vi "ReceiveConnectionStatus.vi"(8 "error in (no error)":errorcluster, 11 "body":variant) -> (0 "error out":errorcluster, 1 "error code":i32, 3 "status":T1, 4 "error info":string)   [LabVIEW 2017, in "ServerComm.lvlib"]
doc: "Returns whether the connection between the device and NI InsightCM Server is online or offline."
uses:
  <vilib>/addons/InsightCM/Devices/Shared/Common/ServerComm/ServerComm.lvlib
  <vilib>/addons/InsightCM/Devices/Shared/Common/ServerComm/controls/ConnectionStatus.ctl
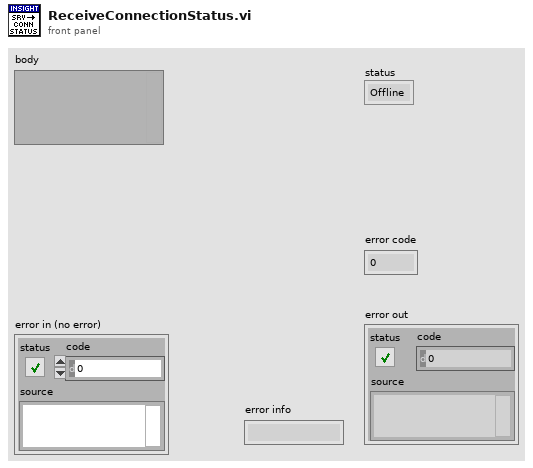
[diagram p1: front panel]
types:
  T1 = typedef "ServerComm.lvlib/ConnectionStatus.ctl" = enum16{"Offline", "NotAuthorized", "Online"}
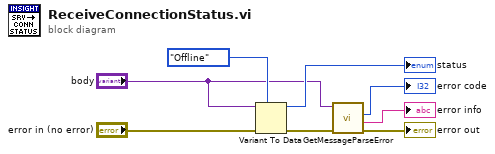
[diagram p0: block diagram]
diagram:
  n1 = Variant To Data(error in="error in (no error)", type=ConnectionStatus."Offline" ("status"), Variant="body") -> (data=→"status":T1, error out=w5:errorcluster)
  n2 = call <vilib>:"GetMessageParseError.vi"("error in (no error)"=w5, "body"="body") -> ("error out"=→"error out":errorcluster, "error info"=→"error info":string, "error code"=→"error code":i32)  [unwired: 7 in]
